vi "bode_atten.vi"() -> ()   [LabVIEW 2014]
doc: "Bode plot ATTEN\nProgramma l'ATF10B per generare un seno con ampiezza e offset scelti\nAcquisiscesia l;inout che la risposta di un circuito\nVaria la frequenza tra FMIN e FMAX e genera il grafico della risposta in funzione della frequenza\nFM & ADL 09-2009, 10/2012\n 10/2013: versione per 8.6"
uses:
  <vilib>/DAQmx/read.llb/DAQmx Read (Analog 1D Wfm NChan NSamp).vi
  <vilib>/Instr/_visa.llb/VISA Configure Serial Port (Instr).vi
  <vilib>/DAQmx/create/channels.llb/DAQmx Create Channel (AI-Voltage-Basic).vi
  <vilib>/DAQmx/configure/timing.llb/DAQmx Timing (Sample Clock).vi
  <vilib>/DAQmx/miscellaneous.llb/DAQmx Fill In Error Info.vi
  <vilib>/measure/matone.llb/Extract Single Tone Information 1 Chan.vi
  <vilib>/Utility/file.llb/Write To Spreadsheet File (DBL).vi
  <vilib>/measure/NI_MAPro.lvlib
  <resource>/objmgr/daqmx.rc
panel:
  in  "Offset (V)":dbl=0.5 min=-10.0 max=10.0 step=0.05
  in  "Ampiezza (V)":dbl=0.5 min=0.01 max=10.0 step=0.05
  in  "FScala Out (CB33)":dbl(ring)=5.0 items=["10"=10.0, "5"=5.0, "0.5"=0.5, "0.05"=0.05]
  out "Frequenza":dbl=9000.0 format="%#_7f"
  out "N. misura":i16=50
  in  "FScala In (CB68)":dbl(ring)=5.0 items=["10"=10.0, "5"=5.0, "0.5"=0.5, "0.05"=0.05]
  in  "F_campionamento (Hz)":dbl=100000.0
  out "Risposta ATF":string="Receive ok\n"
  in  "SALVA I DATI SU FILE":bool=TRUE caption="ON\nOFF"
  out "Fase":cluster{dbl[], dbl[]}(graph)={[100.0, 109.61815804704977, 120.16140573627982, 131.71871965155196, 144.38763428518862, 158.2750651511343, 173.4982110664414, 190.18554321561572, 208.4778893447338, 228.52962223506387, 250.50996248595808, 274.60440660146264, 301.01629243255445, 329.96851518608713, 361.70540848218843, 396.4948063347323, 434.63030345635076, 476.4337329631546, 522.2578823890099, 572.4894709303602, 627.5524130471613, 687.9113959621119, 754.0758012494142, 826.6040036081398, 906.1080830984116, 993.2589906079099, 1088.79221014111, 1193.5139657164482, 1308.3080252526677, 1434.1431588637051, 1572.0813145041684, 1723.2865799613169, 1889.0350068255952, 2070.7253793461787, 2269.891019052065, 2488.212724760281, 2727.5329571745287, 2989.871387780945, 3277.4419432612367, 3592.671489264402, 3938.220311213149, 4317.004564986645, 4732.220886945414, 5187.373370987325, 5686.30314029946, 6233.220763367816, 6832.741787810055, 7489.925691908441, 8210.31858256278, 8999.999999999965], [-3.3665887177852483, -3.700123226448113, -4.028118062790128, -4.4281673855003305, -4.830321725701623, -5.294622725946937, -5.768359970229511, -6.352601264586838, -6.950610748626104, -7.654010983134981, -8.370246017138356, -9.154354356501699, -9.991090016023662, -10.944641260650087, -11.962971259135287, -13.040753260052696, -14.264684576322452, -15.537744545515892, -16.93627096290095, -18.4443118824162, -20.083995187706194, -21.79731308113321, -23.62180164592729, -25.57373618604504, -27.601405485014936, -29.737921321438762, -31.963459773455156, -34.24969024498253, -36.57187792514435, -38.94063777108295, -41.29645876834843, -43.6550655750593, -45.96311073921197, -48.22478948324985, -50.37119719567454, -52.407748921554386, -54.333607142636936, -56.12645716441807, -57.72107146098617, -59.18140055965944, -60.44248430535988, -61.53284746858367, -62.476592446911056, -63.182861181812825, -63.718892450621, -64.04313048803937, -64.19408276209815, -64.15192658058876, -63.871050137156374, -63.43031992247117]}
  out "GAIN":cluster{dbl[], dbl[]}(graph)={[100.0, 109.61815804704977, 120.16140573627982, 131.71871965155196, 144.38763428518862, 158.2750651511343, 173.4982110664414, 190.18554321561572, 208.4778893447338, 228.52962223506387, 250.50996248595808, 274.60440660146264, 301.01629243255445, 329.96851518608713, 361.70540848218843, 396.4948063347323, 434.63030345635076, 476.4337329631546, 522.2578823890099, 572.4894709303602, 627.5524130471613, 687.9113959621119, 754.0758012494142, 826.6040036081398, 906.1080830984116, 993.2589906079099, 1088.79221014111, 1193.5139657164482, 1308.3080252526677, 1434.1431588637051, 1572.0813145041684, 1723.2865799613169, 1889.0350068255952, 2070.7253793461787, 2269.891019052065, 2488.212724760281, 2727.5329571745287, 2989.871387780945, 3277.4419432612367, 3592.671489264402, 3938.220311213149, 4317.004564986645, 4732.220886945414, 5187.373370987325, 5686.30314029946, 6233.220763367816, 6832.741787810055, 7489.925691908441, 8210.31858256278, 8999.999999999965], [0.9977934611714828, 0.9973942841893607, 0.9969514449456482, 0.9963647964208311, 0.9957226050730295, 0.9949942010150018, 0.9940628611709184, 0.9928253202745592, 0.9915293490191036, 0.9897392988118141, 0.9878505109010701, 0.9854699589308881, 0.9827297447292448, 0.9794197865298515, 0.9754334507989486, 0.9709014043514924, 0.9652267747196113, 0.9588953223887673, 0.9512651029901658, 0.9424056583239725, 0.9317427524144849, 0.9197578833646268, 0.9058879545356355, 0.8898491112859954, 0.8718920649501838, 0.8516645346538394, 0.8290000350185601, 0.8040870556696726, 0.7771192251435036, 0.7478113943007981, 0.7166776137577737, 0.684033333682016, 0.6501668070722814, 0.6153182636776587, 0.5800687308324993, 0.5448614520591276, 0.5098720426005084, 0.47578904474596667, 0.4425900372872962, 0.4104720959012425, 0.3799444211411506, 0.3508941286835518, 0.3236252730694512, 0.2978329636149937, 0.2737248235070636, 0.25121504944313877, 0.23038101385968812, 0.21113646995201163, 0.19339222639151807, 0.17698358760477434]}
  out "Vout (bianco) Vin (giallo)":waveform(dbl)[](graph)=[{"t0"=timestamp(3416385464.414006 s since 1904-01-01), "dt"=9.999999999999972e-06, "Y"=array[10000 elements], "attributes"=variant("NI_ChannelName"=variant(string "Dev1/ai0"), "NI_UnitDescription"=variant(string "Volts"))}, {"t0"=timestamp(3416385464.414011 s since 1904-01-01), "dt"=9.999999999999972e-06, "Y"=array[10000 elements], "attributes"=variant("NI_ChannelName"=variant(string "Dev1/ai1"), "NI_UnitDescription"=variant(string "Volts"))}]
  in  "Numero misure":i16=50
  in  "Freqmax":dbl=9000.0 min=0.0 max=100000.0
  in  "Freqmin":dbl=100.0 min=0.0 max=100000.0
  # "Primo passo: scegliere frequenza di campionamento, fondo scala canali\nSecondo passo: scegliere l'intervallo di frequenza e il numero di misure\nTerzo passo: impostare ampiezza e offset del generatore\nQuarto passo: scegliere se salvare i dati sul file\nQuinto passo: premere la freccia bianca"
  # "Foma d'onda generata Vin(t)"
  # "I Collegamenti"
  # "I due canali di misura (riferiti a terra) sono il CB68 (Vin) e CB33 (Vout).\nLa terra del circuito e quella del generatore DEVONO essere in comune alla terra della scheda (CB29)."
  # "NO\nSI"
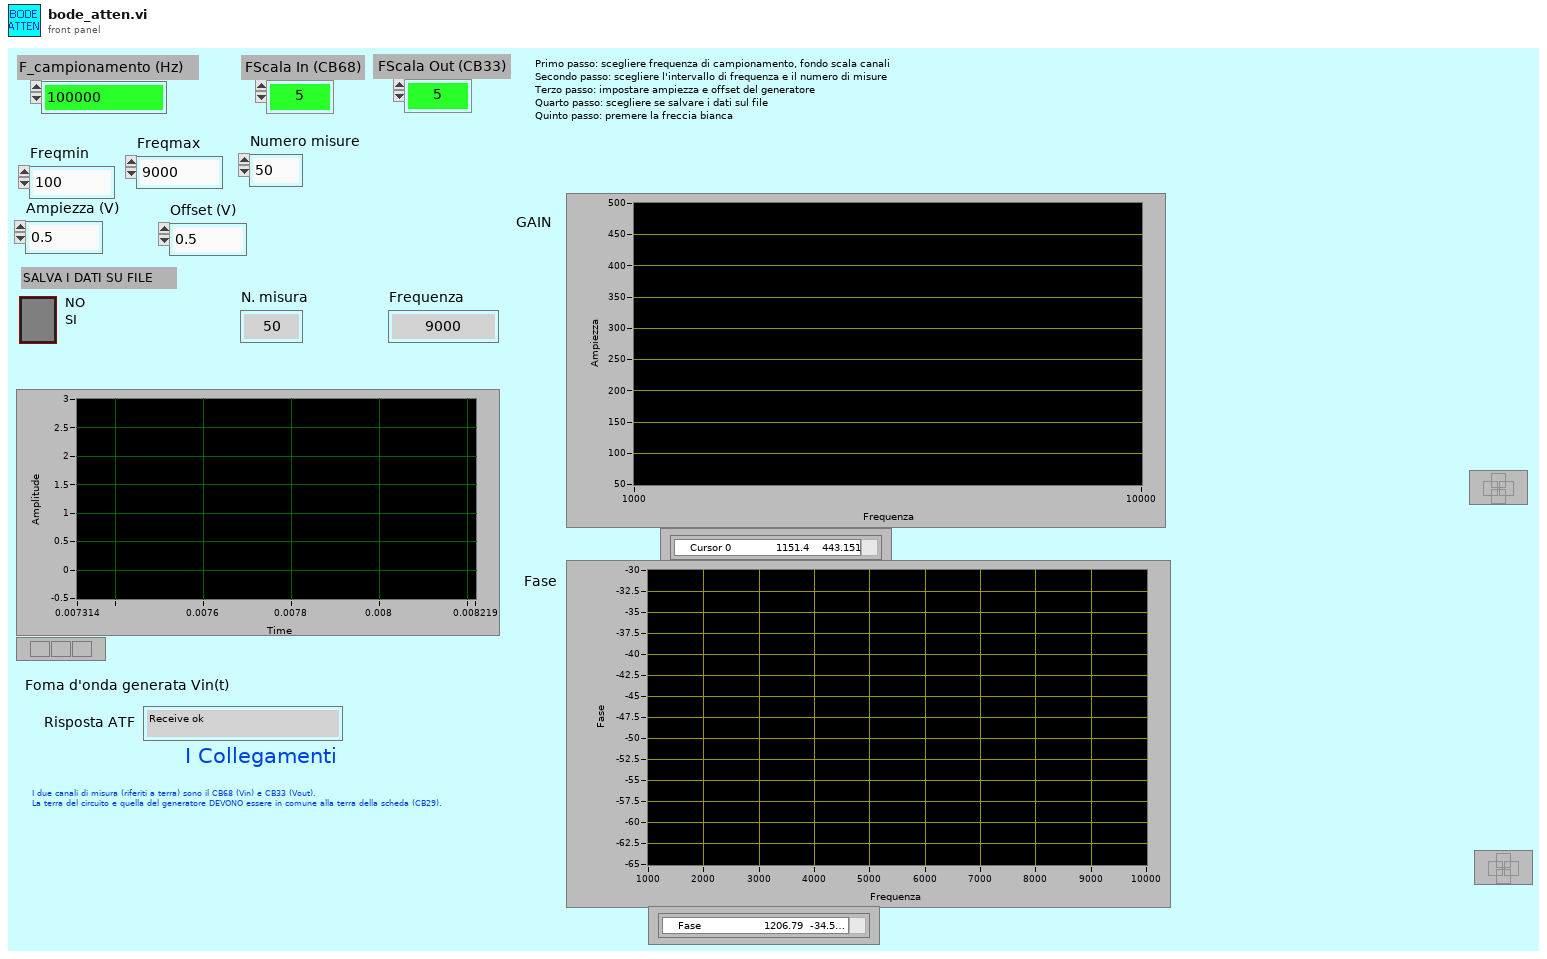
[diagram p1: front panel]
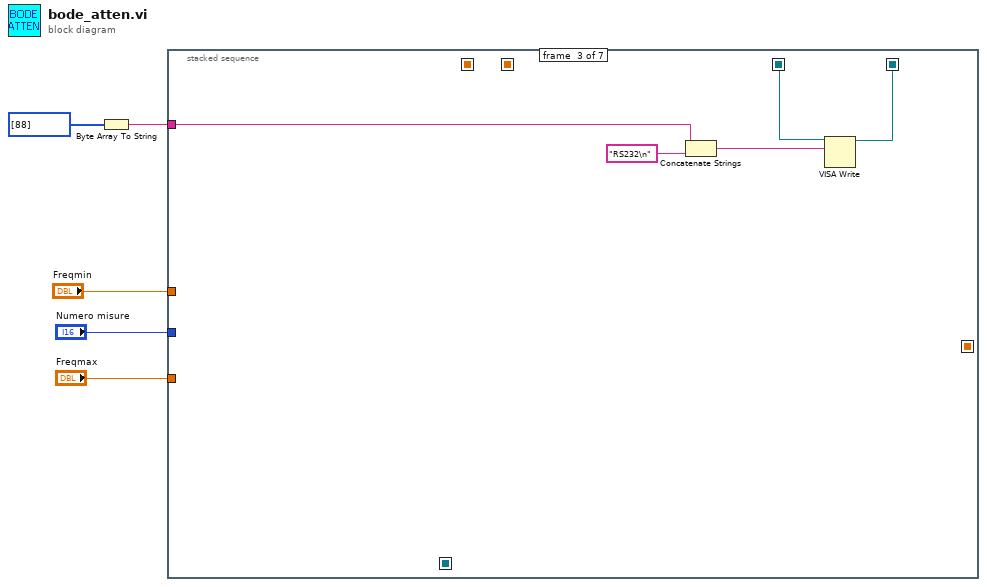
[diagram p0: block diagram]
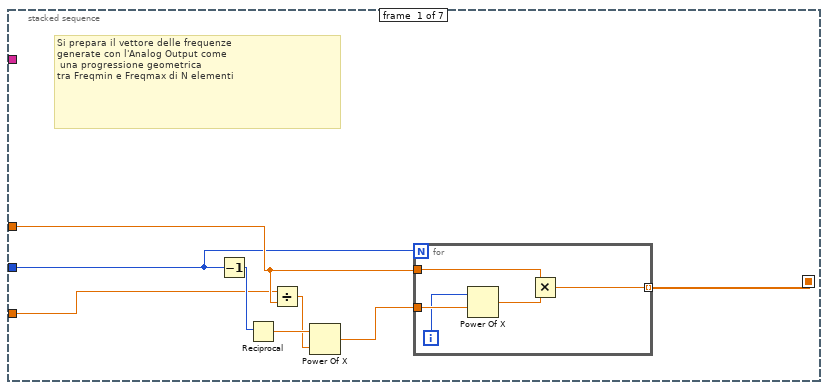
[diagram p2: hidden frame]
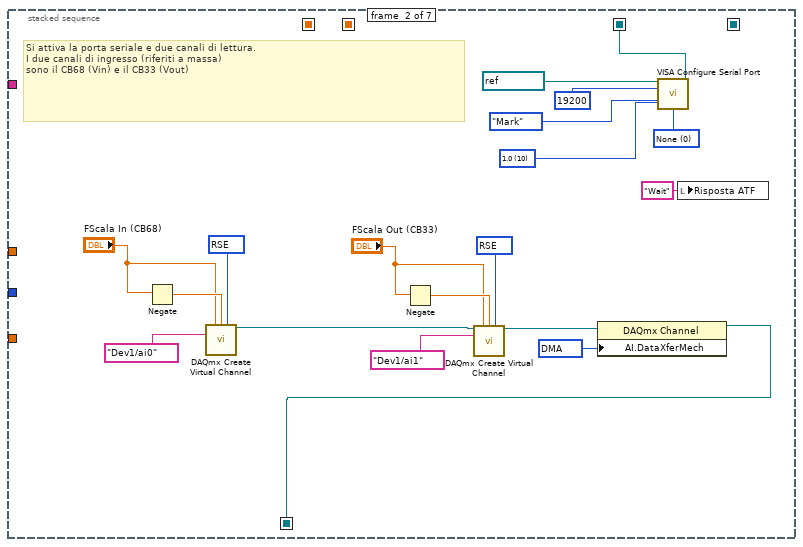
[diagram p3: hidden frame]
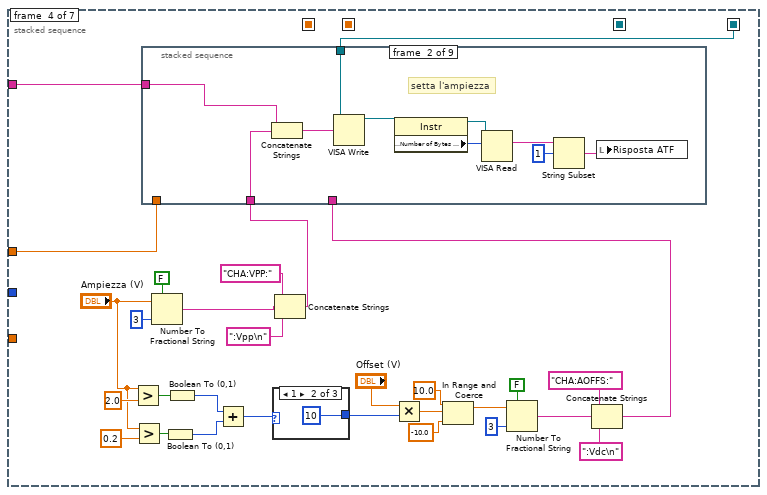
[diagram p4: hidden frame]
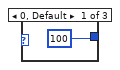
[diagram p5: hidden frame]
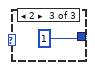
[diagram p6: hidden frame]
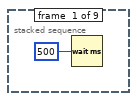
[diagram p7: hidden frame]
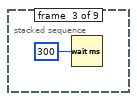
[diagram p8: hidden frame]
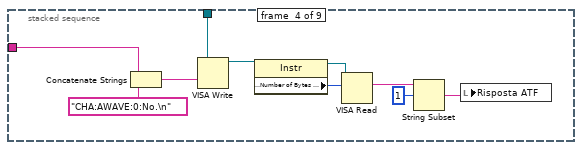
[diagram p9: hidden frame]
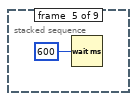
[diagram p10: hidden frame]
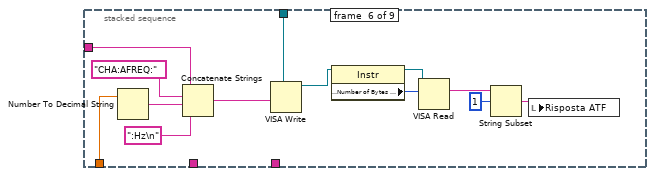
[diagram p11: hidden frame]
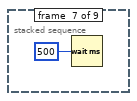
[diagram p12: hidden frame]
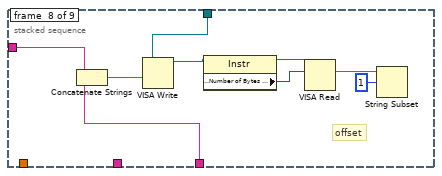
[diagram p13: hidden frame]
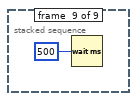
[diagram p14: hidden frame]
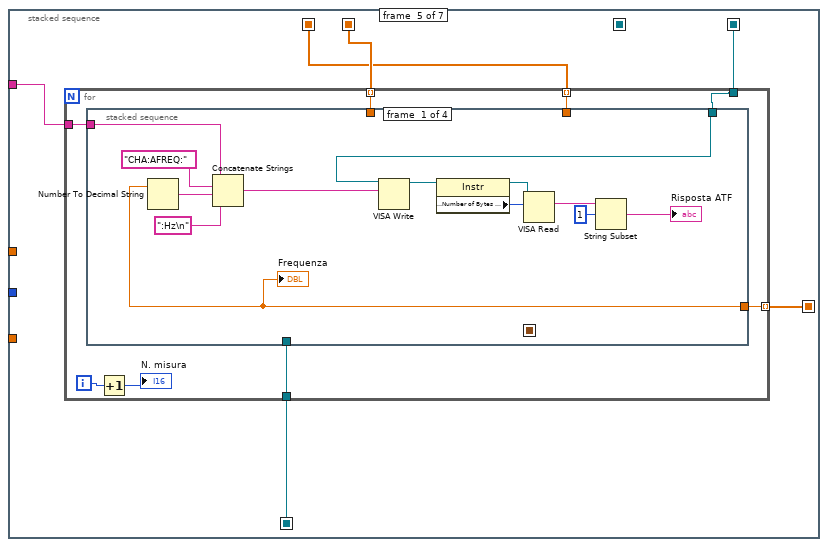
[diagram p15: hidden frame]
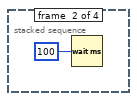
[diagram p16: hidden frame]
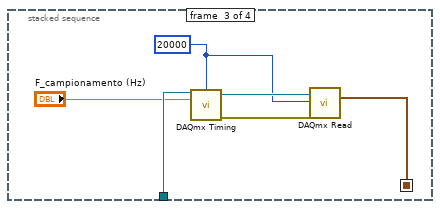
[diagram p17: hidden frame]
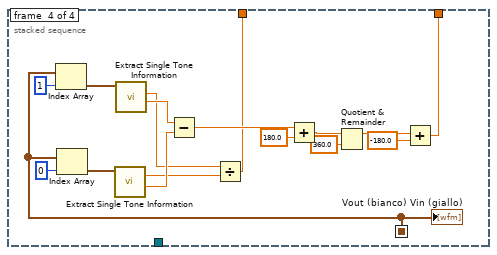
[diagram p18: hidden frame]
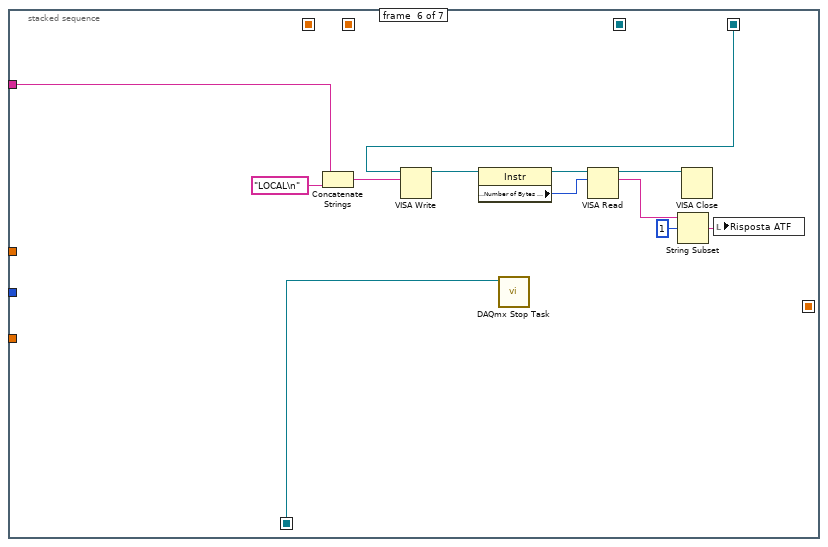
[diagram p19: hidden frame]
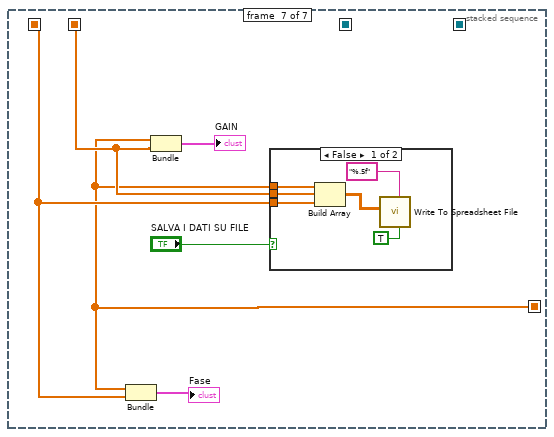
[diagram p20: hidden frame]
diagram:
  n1 = Byte Array To String(unsigned byte array=u8[] [88] ("INDIRIZZO")) -> (string=w1:string)
  n2 = stacked-sequence {
    seq-local: [w6 _ _ _ _ _ _] -> [_ _ _ _ w126 _ w185]
    seq-local: [_ w25 _ _ _ _ _] -> [_ _ _ _ w127 w184 _]
    seq-local: [_ _ _ _ w123 _ _] -> [_ _ _ _ _ _ w188]
    seq-local: [_ _ _ _ w122 _ _] -> [_ _ _ _ _ _ w187]
    seq-local: [_ w31 _ _ _ _ _] -> [_ _ w40 _ _ _ _]
    seq-local: [_ _ w39 _ _ _ _] -> [_ _ _ w70 w125 w181 _]
    tunnel: "Freqmin" -> [w9 _ _ w69 _ _ _]
    tunnel: "Numero misure" -> [w8 _ _ _ _ _ _]
    tunnel: "Freqmax" -> [w7 _ _ _ _ _ _]
    tunnel: w1 -> [_ _ w38 w71 w124 w173 _]
    frame #0 {
      # "Si prepara il vettore delle frequenze\ngenerate con l'Analog Output come\n una progressione geometrica\ntra Freqmin e Freqmax di N elementi"
      n3 = Decrement(x=w8) -> (x-1=w13:i16)
      n4 = Reciprocal(x=w13) -> (1/x=w12:dbl)
      n5 = Divide(x=w7, y=w9) -> (x/y=w11:dbl)
      n6 = Power Of X(1:w11, 2:w12) -> (0:w10:dbl)
      n7 = for {
        N: w8 -> [_]
        tunnel: w10 -> [w18]
        tunnel: w9 -> [w16]
        tunnel: [w14] -> w6 mode=indexing
        i -> [w17]
        n8 = Power Of X(1:w18, 2:w17) -> (0:w15:dbl)
        n9 = Multiply(x=w16, y=w15) -> (x*y=w14:dbl)
      }
    }
    frame #1 {
      w24 = 10054 items=["DMA"=10054, "Interrupts"=10204, "Programmed I/O"=10264, "USB Bulk"=12590] ("AI.DataXferMech")
      w28 = 10083 items=["default"=-1, "RSE"=10083, "NRSE"=10078, "Differential"=10106, "Pseudodifferential"=12529] ("input terminal configuration")
      w33 = u16 10 items=["1.0"=10, "1.5"=15, "2.0"=20] ("stop bits")
      w32 = u16 0 items=["None", "XON/XOFF", "RTS/CTS", "XON/XOFF & RTS/CTS", "DTR/DSR", "XON/XOFF & DTR/DSR"] ("flow control (0:none)")
      w36 = 10083 items=["default"=-1, "RSE"=10083, "NRSE"=10078, "Differential"=10106, "Pseudodifferential"=12529] ("input terminal configuration")
      # "Si attiva la porta seriale e due canali di lettura.\nI due canali di ingresso (riferiti a massa)\nsono il CB68 (Vin) e il CB33 (Vout)"
      n10 = Negate(x="FScala In (CB68)") -> (-x=w23:dbl)
      n11 = call-poly <vilib>:"DAQmx Create Virtual Channel.vi"("maximum value"="FScala In (CB68)", "minimum value"=w23, "input terminal configuration"=w36, "physical channels"=tag "Dev1/ai0") -> ("task out"=w27:refnum<k21>)  [unwired: 5 in, 6 out]
      n12 = Negate(x="FScala Out (CB33)") -> (-x=w21:dbl)
      n13 = call-poly <vilib>:"DAQmx Create Virtual Channel.vi"("task in"=w27, "maximum value"="FScala Out (CB33)", "minimum value"=w21, "input terminal configuration"=w28, "physical channels"=tag "Dev1/ai1") -> ("task out"=w26:refnum<k21>)  [unwired: 4 in, 6 out]
      n14 = property class="DAQmx Channel"(reference=w26, "AI.DataXferMech"=w24) -> (reference out=w25:refnum<k21>)  [unwired: 1 in, 1 out]
      n15 = call-poly "VISA Configure Serial Port"("VISA resource name"=refnum<visa-resource-name> "COM1", "baud rate (9600)"=u32 19200, "parity (0:none)"=enum16{"None", "Odd", "Even", "Mark", "Space"}."Mark" ("parity"), "stop bits (10: 1 bit)"=w33, "flow control (0:none)"=w32) -> ("VISA resource name out"=w31:refnum<visa-resource-name>)  [unwired: 2 in, 8 out]
      n16 = local write "Risposta ATF"("Wait" ("Risposta ATF")) -> ()
    }
    frame #2 {
      n17 = Concatenate Strings(w38, "RS232\n" ("write buffer")) -> (w41:string)
      n18 = VISA Write(VISA resource name=w40, write buffer=w41) -> (VISA resource name out=w39:refnum<visa-resource-name>)  [unwired: 1 in, 2 out]
    }
    frame #3 {
      n19 = Greater?(x="Ampiezza (V)", y=2.0) -> (0:w59:bool)
      n20 = Greater?(x="Ampiezza (V)", y=0.2) -> (0:w58:bool)
      n21 = Number To Fractional String(use system decimal point (T)=FALSE, number="Ampiezza (V)", precision (6)=i16 3) -> (F-format string=w64:string)  [unwired: 1 out]
      n22 = Boolean To (0,1)(Boolean=w58) -> (0, 1=w56:i16)
      n23 = Boolean To (0,1)(Boolean=w59) -> (0, 1=w57:i16)
      n24 = Add(x=w57, y=w56) -> (x+y=w55:i16)
      n25 = case shown="1" w55 {
        tunnel: [100 10 1] -> w54
        frame 0, Default {
        }
        frame 1 {
        }
        frame 2 {
        }
      }
      n26 = Concatenate Strings("CHA:VPP:" ("write buffer"), w64, ":Vpp\n" ("write buffer")) -> (w63:string)
      n27 = Multiply(x="Offset (V)", y=w54) -> (x*y=w52:dbl)
      n28 = In Range and Coerce(upper limit=10.0, x=w52, lower limit=-10.0) -> (coerced(x)=w45:dbl)  [unwired: 1 out]
      n29 = Number To Fractional String(use system decimal point (T)=FALSE, number=w45, precision (6)=i16 3) -> (F-format string=w44:string)  [unwired: 1 out]
      n30 = Concatenate Strings("CHA:AOFFS:" ("write buffer"), w44, ":Vdc\n" ("write buffer")) -> (w43:string)
      n31 = stacked-sequence {
        tunnel: w71 -> [_ w84 _ w94 _ w105 _ w119 _]
        tunnel: w70 -> [_ w83 _ w93 _ w104 _ w118 _]
        tunnel: w69 -> [_ _ _ _ _ w106 _ _ _]
        tunnel: w63 -> [_ w76 _ _ _ _ _ _ _]
        tunnel: w43 -> [_ _ _ _ _ _ _ w112 _]
        frame #0 {
          n32 = Wait (ms)(milliseconds to wait=u32 500 ("millisecond multiple")) -> ()  [unwired: 1 out]
        }
        frame #1 {
          # "setta l'ampiezza"
          n33 = Concatenate Strings(w84, w76) -> (w85:string)
          n34 = VISA Write(VISA resource name=w83, write buffer=w85) -> (VISA resource name out=w78:refnum<visa-resource-name>)  [unwired: 1 in, 2 out]
          n35 = property class="Instr"(reference=w78) -> (reference out=w82:refnum<visa-resource-name>, "Serial Settings:Number of Bytes at Serial Port"=w81:u32)  [unwired: 1 in, 1 out]
          n36 = VISA Read(VISA resource name=w82, byte count=w81) -> (read buffer=w80:string)  [unwired: 1 in, 3 out]
          n37 = String Subset(string=w80, offset (0)=1) -> (substring=w77:string)  [unwired: 1 out]
          n38 = local write "Risposta ATF"(w77) -> ()
        }
        frame #2 {
          n39 = Wait (ms)(milliseconds to wait=u32 300 ("millisecond multiple")) -> ()  [unwired: 1 out]
        }
        frame #3 {
          n40 = Concatenate Strings(w94, "CHA:AWAVE:0:No.\n" ("write buffer")) -> (w96:string)
          n41 = VISA Write(VISA resource name=w93, write buffer=w96) -> (VISA resource name out=w88:refnum<visa-resource-name>)  [unwired: 1 in, 2 out]
          n42 = property class="Instr"(reference=w88) -> (reference out=w92:refnum<visa-resource-name>, "Serial Settings:Number of Bytes at Serial Port"=w91:u32)  [unwired: 1 in, 1 out]
          n43 = VISA Read(VISA resource name=w92, byte count=w91) -> (read buffer=w90:string)  [unwired: 1 in, 3 out]
          n44 = String Subset(string=w90, offset (0)=1) -> (substring=w87:string)  [unwired: 1 out]
          n45 = local write "Risposta ATF"(w87) -> ()
        }
        frame #4 {
          n46 = Wait (ms)(milliseconds to wait=u32 600 ("millisecond multiple")) -> ()  [unwired: 1 out]
        }
        frame #5 {
          n47 = Number To Decimal String(number=w106) -> (decimal integer string=w109:string)  [unwired: 1 out]
          n48 = Concatenate Strings(w105, "CHA:AFREQ:" ("string"), w109, ":Hz\n") -> (w107:string)
          n49 = VISA Write(VISA resource name=w104, write buffer=w107) -> (VISA resource name out=w98:refnum<visa-resource-name>)  [unwired: 1 in, 2 out]
          n50 = property class="Instr"(reference=w98) -> (reference out=w99:refnum<visa-resource-name>, "Serial Settings:Number of Bytes at Serial Port"=w100:u32)  [unwired: 1 in, 1 out]
          n51 = VISA Read(VISA resource name=w99, byte count=w100) -> (read buffer=w101:string)  [unwired: 1 in, 3 out]
          n52 = String Subset(string=w101, offset (0)=1) -> (substring=w103:string)  [unwired: 1 out]
          n53 = local write "Risposta ATF"(w103) -> ()
        }
        frame #6 {
          n54 = Wait (ms)(milliseconds to wait=u32 500 ("millisecond multiple")) -> ()  [unwired: 1 out]
        }
        frame #7 {
          # "offset"
          n55 = Concatenate Strings(w119, w112) -> (w120:string)
          n56 = VISA Write(VISA resource name=w118, write buffer=w120) -> (VISA resource name out=w115:refnum<visa-resource-name>)  [unwired: 1 in, 2 out]
          n57 = property class="Instr"(reference=w115) -> (reference out=w114:refnum<visa-resource-name>, "Serial Settings:Number of Bytes at Serial Port"=w113:u32)  [unwired: 1 in, 1 out]
          n58 = VISA Read(VISA resource name=w114, byte count=w113) -> (read buffer=w117:string)  [unwired: 1 in, 3 out]
          n59 = String Subset(string=w117, offset (0)=1) -> ()  [unwired: 2 out]
        }
        frame #8 {
          n60 = Wait (ms)(milliseconds to wait=u32 500 ("millisecond multiple")) -> ()  [unwired: 1 out]
        }
      }
    }
    frame #4 {
      n61 = for {
        tunnel: w126 -> [w135] mode=indexing
        tunnel: w127 -> [w134]
        tunnel: w125 -> [w128]
        tunnel: w124 -> [w133]
        tunnel: [w132] -> w123 mode=indexing
        tunnel: [w131] -> w122 mode=indexing
        i -> [w130]
        n62 = stacked-sequence {
          seq-local: [_ _ w153 _] -> [_ _ _ w170]
          tunnel: w135 -> [w136 _ _ _]
          tunnel: w134 -> [_ _ w152 _]
          tunnel: w128 -> [w145 _ _ _]
          tunnel: w133 -> [w141 _ _ _]
          tunnel: [_ _ _ w157] -> w132
          tunnel: [_ _ _ w156] -> w131
          frame #0 {
            n63 = Number To Decimal String(number=w136) -> (decimal integer string=w139:string)  [unwired: 1 out]
            n64 = Concatenate Strings(w141, "CHA:AFREQ:" ("string"), w139, ":Hz\n") -> (w137:string)
            n65 = VISA Write(VISA resource name=w145, write buffer=w137) -> (VISA resource name out=w148:refnum<visa-resource-name>)  [unwired: 1 in, 2 out]
            n66 = property class="Instr"(reference=w148) -> (reference out=w147:refnum<visa-resource-name>, "Serial Settings:Number of Bytes at Serial Port"=w146:u32)  [unwired: 1 in, 1 out]
            n67 = VISA Read(VISA resource name=w147, byte count=w146) -> (read buffer=w144:string)  [unwired: 1 in, 3 out]
            n68 = String Subset(string=w144, offset (0)=1) -> (substring=→"Risposta ATF":string)  [unwired: 1 out]
            "Frequenza" <- w136
          }
          frame #1 {
            n69 = Wait (ms)(milliseconds to wait=u32 100 ("millisecond multiple")) -> ()  [unwired: 1 out]
          }
          frame #2 {
            w150 = 20000 ("samples per channel")
            n70 = call-poly <vilib>:"DAQmx Timing.vi"("task/channels in"=w152, "samples per channel"=w150, "rate"="F_campionamento (Hz)") -> ("task out"=w155:refnum<k21>, "error out"=w154:errorcluster)  [unwired: 4 in, 7 out]
            n71 = call-poly <vilib>:"DAQmx Read.vi"("task/channels in"=w155, "number of samples per channel"=w150, "error in"=w154) -> ("data"=w153:waveform(dbl)[])  [unwired: 12 out]
          }
          frame #3 {
            n72 = Index Array(array=w170, index=1) -> (element=w171:waveform(dbl))
            n73 = Index Array(array=w170, index=0) -> (element=w172:waveform(dbl))
            n74 = call-poly <vilib>:"Extract Single Tone Information.vi"("time signal in"=w172) -> ("detected phase (deg)"=w167:dbl, "detected amplitude"=w164:dbl)  [unwired: 3 in, 6 out]
            n75 = call-poly <vilib>:"Extract Single Tone Information.vi"("time signal in"=w171) -> ("detected phase (deg)"=w168:dbl, "detected amplitude"=w165:dbl)  [unwired: 3 in, 6 out]
            n76 = Subtract(x=w168, y=w167) -> (x-y=w158:dbl)
            n77 = Divide(x=w165, y=w164) -> (x/y=w157:dbl)
            n78 = Add(x=w158, y=180.0) -> (x+y=w160:dbl)
            n79 = Quotient & Remainder(x=w160, y=360.0) -> (x-y*floor(x/y)=w162:dbl)  [unwired: 1 out]
            n80 = Add(x=w162, y=-180.0) -> (x+y=w156:dbl)
            "Vout (bianco) Vin (giallo)" <- w170
          }
        }
        n81 = Increment(x=w130) -> (x+1=→"N. misura":i32)
      }
    }
    frame #5 {
      n82 = Concatenate Strings(w173, "LOCAL\n" ("write buffer")) -> (w182:string)
      n83 = VISA Write(VISA resource name=w181, write buffer=w182) -> (VISA resource name out=w180:refnum<visa-resource-name>)  [unwired: 1 in, 2 out]
      n84 = property class="Instr"(reference=w180) -> (reference out=w179:refnum<visa-resource-name>, "Serial Settings:Number of Bytes at Serial Port"=w177:u32)  [unwired: 1 in, 1 out]
      n85 = call <vilib>:"DAQmx Stop Task.vi"("task/channels in"=w184) -> ()  [unwired: 1 in, 14 out]
      n86 = VISA Read(VISA resource name=w179, byte count=w177) -> (VISA resource name out=w178:refnum<visa-resource-name>, read buffer=w175:string)  [unwired: 1 in, 2 out]
      n87 = String Subset(string=w175, offset (0)=1) -> (substring=w174:string)  [unwired: 1 out]
      n88 = VISA Close(VISA resource name=w178) -> ()  [unwired: 1 in, 1 out]
      n89 = local write "Risposta ATF"(w174) -> ()
    }
    frame #6 {
      n90 = Bundle(w185, w187) -> (→"Fase":cluster{dbl[], dbl[]})  [unwired: 1 out]
      n91 = Bundle(w185, w188) -> (→"GAIN":cluster{dbl[], dbl[]})  [unwired: 1 out]
      n92 = case shown="False" "SALVA I DATI SU FILE" {
        tunnel: w185 -> [w196 _]
        tunnel: w188 -> [w195 _]
        tunnel: w187 -> [w194 _]
        frame False {
          n93 = Build Array(w196, w195, w194) -> (w193:dbl[][])
          n94 = call-poly <vilib>:"Write To Spreadsheet File.vi"("transpose? (no:F)"=TRUE, "format (%.3f)"="%.5f", "2D data"=w193) -> ()  [unwired: 3 in, 3 out]
        }
        frame True {
        }
      }
    }
  }
